vi "EZ1 MB1010 Sonar - Analog.vi"(7 "Enum":T3, 9 "Scaling factor (V/in)":dbl=0.009585, 10 "Samples Per Second":dbl=1000.0, 11 "Average Bits":u8=3 max=15) -> (0 "error out":errorcluster, 3 "distance":dbl(slide)=255.4405658841941 scale=0.0..250.0 scale format="%3d")   [LabVIEW 2013]
doc: "This example shows how to use the MaxBotix LV-MaxSonar-EZ1 Sonar Range Finder MB1010. It will display the distance from the sensor in inches.\n\nThis example works with the NI 9201 module with an Analog Breakout attached. The Analog Breakout should have 12V applied to the WAGO connector (J3). The sensor is attached to the 3x8 header using a 3-pin PWM connector."
uses:
  Sonar Read Control.ctl
  <vilib>/Rock Robotics/SystemInterfaces/AI/FPGA_AIChannel.ctl
  <vilib>/Rock Robotics/SystemInterfaces/Typedef/FPGA_TypedefAnalogModule.ctl
panel:
  in  "Analog Module 2":T1
  in  "Channel 2":T2
  # "Set these inputs before running."
  # "These can be set while running."
  # "Wiring Diagram for Analog Breakout connected to an NI 9201"
  # "EZ1 MB1010"
  # "This shows wiring for a MaxBotix LV-MaxSonar-EZ1 Sonar Range Finder MB1010."
  # "GND"
  # "+5"
  # "TX"
  # "RX"
  # "AN"
  # "PW"
  # "BW"
  # "jumper to read battery or AI8"
  # "GND"
  # "SIG"
  # "5V"
  # "AI8\nAI7\nAI6\nAI5\nAI4\nAI3\nAI2\nAI1"
  # "+"
  # "12V from battery"
  # "-"
  # "\"power good\" LED"
  # "Output information."
  # "EZ1"
  # "inches"
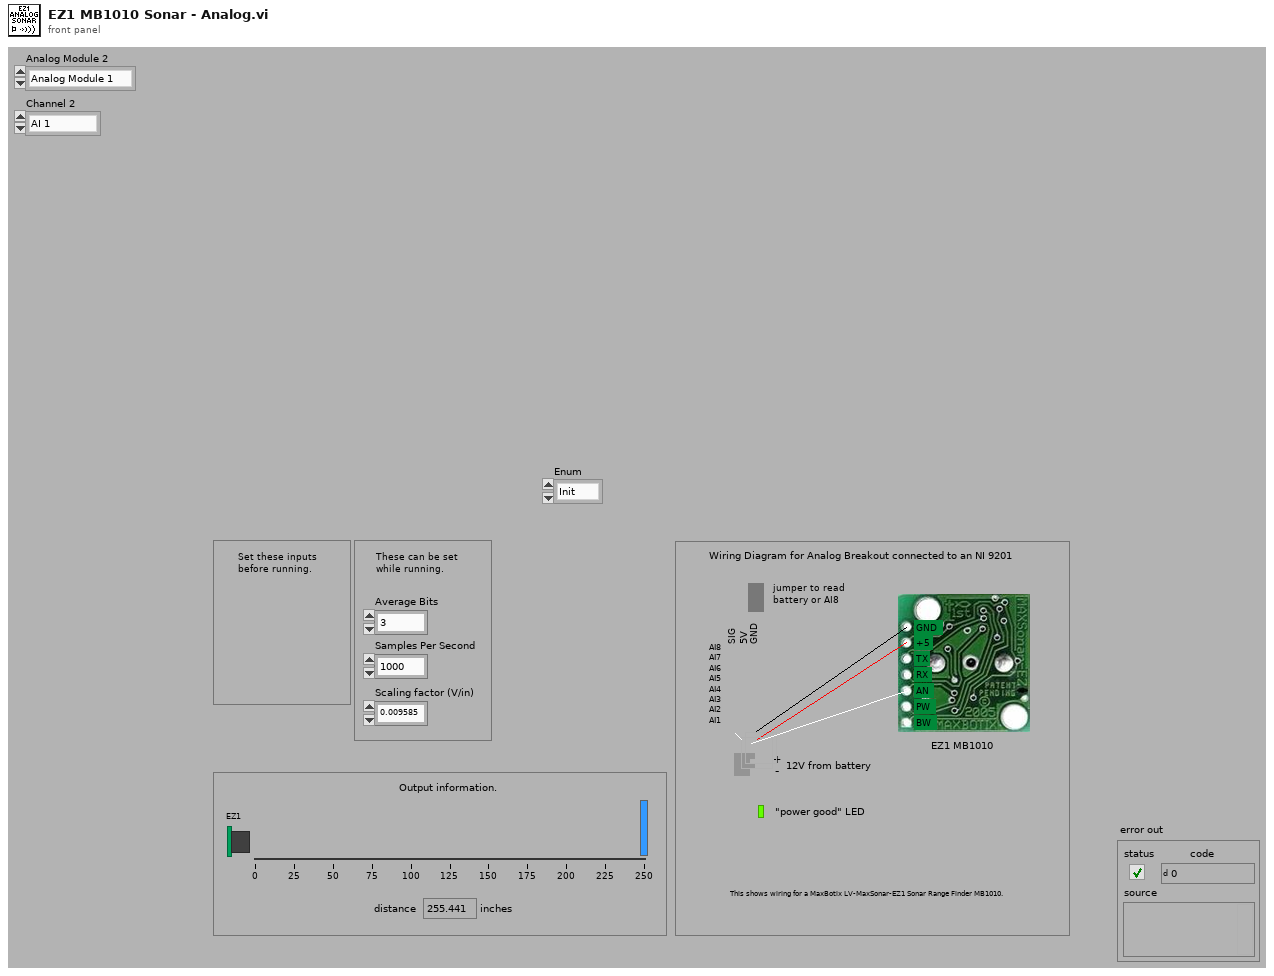
[diagram p1: front panel]
types:
  T1 = typedef "FPGA_TypedefAnalogModule.ctl" = enum16{"Analog Module 1", "Analog Module 2"}
  T2 = typedef "FPGA_AIChannel.ctl" = enum8{"AI 1", "AI 2", "AI 3", "AI 4", "AI 5", "AI 6", "AI 7", "AI 8", "Invalid"}
  T3 = typedef "Sonar Read Control.ctl" = enum16{"Init", "ReadValue", "Disable"}
  T4 = typedef "WPI_AnalogChannelDevRef.ctl" = cluster{"DevStatus":errorcluster, "Analog Module":T1, "Analog Channel":T2}
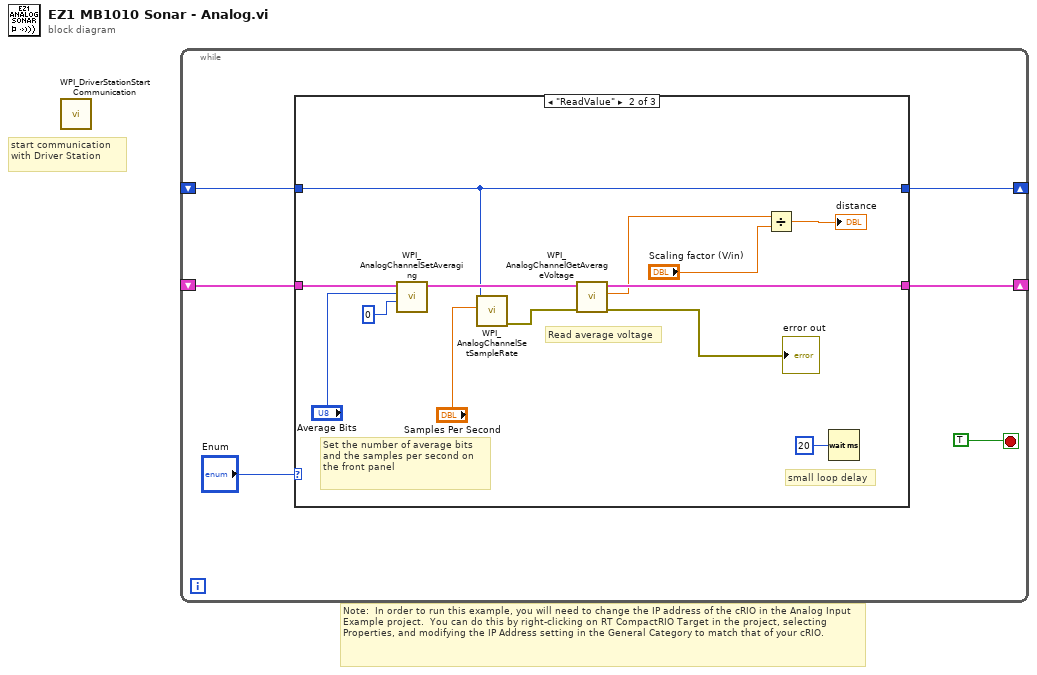
[diagram p0: block diagram]
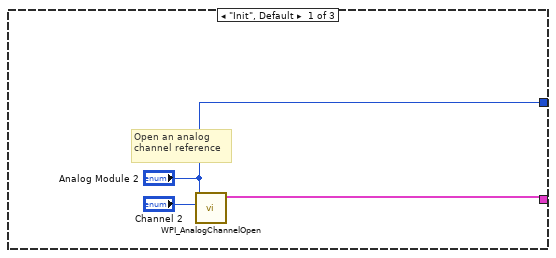
[diagram p2: hidden frame]
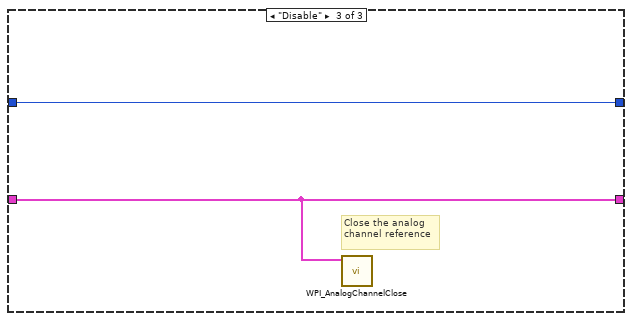
[diagram p3: hidden frame]
diagram:
  # "start communication with Driver Station"
  # "Note:  In order to run this example, you will need to change the IP address of the cRIO in the Analog Input Example project.  You can do this by right-clicking on RT CompactRIO Target in the project, selecting Properties, and modifying the IP Address setting in the General Category to match that of your cRIO."
  n1 = call <vilib>:"WPI_DriverStationStart Communication.vi"() -> ()  [unwired: 1 in, 11 out]
  n2 = while {
    shift-right: [w6] -> _
    shift-left: _ -> [w5]
    shift-right: [w2] -> _
    shift-left: _ -> [w4]
    stop <- TRUE stop-if-true
    n3 = case shown="\"ReadValue\"" "Enum" {
      tunnel: [w7 w22 w23] -> w6
      tunnel: w5 -> [_ w20 w23]
      tunnel: w4 -> [_ w11 w24]
      tunnel: ["Analog Module 2" w11 w24] -> w2
      frame "Init", Default {
        # "Open an analog channel reference"
        n4 = call <vilib>:"WPI_AnalogChannelOpen.vi"("Analog Channel"="Channel 2", "Analog Module (Module 1)"="Analog Module 2") -> ("AIDeviceRef"=w7:T4)  [unwired: 1 in, 8 out]
      }
      frame "ReadValue" {
        # "small loop delay"
        # "Read average voltage"
        # "Set the number of average bits and the samples per second on the front panel"
        n5 = call <vilib>:"WPI_AnalogChannelSetAveraging.vi"("OversampleBits"=u8 0, "AverageBits"="Average Bits", "AIDeviceRef"=w20) -> ("AIDeviceRef"=w13:T4)  [unwired: 1 in, 7 out]
        n6 = call <vilib>:"WPI_AnalogChannelSetSampleRate.vi"("Samples Per Second"="Samples Per Second", "Analog Module (Module 1)"=w11) -> ("error out"=w12:errorcluster)  [unwired: 2 in, 7 out]
        n7 = call <vilib>:"WPI_AnalogChannelGetAverageVoltage.vi"("error in (no error)"=w12, "AIDeviceRef"=w13) -> ("error out"=→"error out":errorcluster, "Voltage"=w15:dbl, "AIDeviceRef"=w22:T4)  [unwired: 7 out]
        n8 = Divide(x=w15, y="Scaling factor (V/in)") -> (x/y=→"distance":dbl)
        n9 = Wait (ms)(milliseconds to wait=u32 20) -> ()  [unwired: 1 out]
      }
      frame "Disable" {
        # "Close the analog\nchannel reference"
        n10 = call <vilib>:"WPI_AnalogChannelClose.vi"("AIDeviceRef"=w23) -> ()  [unwired: 1 in, 10 out]
      }
    }
  }
